vi "Fieldbus Read_Write.vi"(8 "error in (no error)":errorcluster, 11 "FHPP in":refnum<class "FHPP.lvclass">) -> (0 "error out":errorcluster, 3 "FHPP out":refnum<class "FHPP.lvclass">)   [LabVIEW 2022 SP3, in "FHPP.lvclass"]
uses:
  FHPP.lvclass
  FHPP.lvclass/FHPP.ctl
  <vilib>/Modbus/master/Modbus Master.lvclass
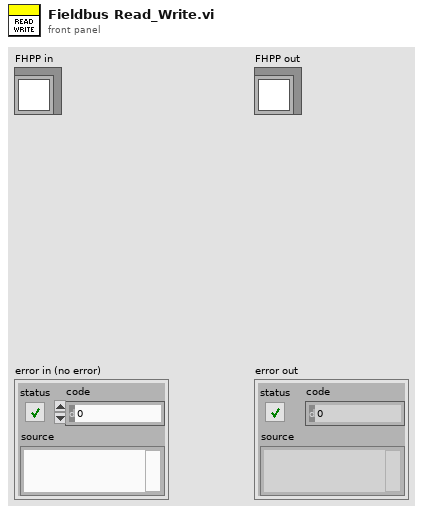
[diagram p1: front panel]
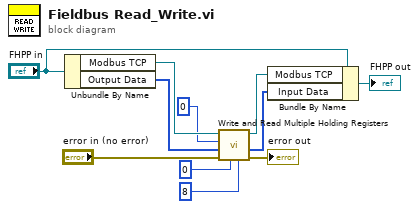
[diagram p0: block diagram]
diagram:
  n1 = Unbundle By Name("FHPP in") -> ("Modbus TCP"=w8:refnum<class "Modbus Master.lvclass">, "Output Data"=w7:u16[])
  n2 = call-dynamic "Write and Read Multiple Holding Registers.vi"("read count"=u16 8 ("number of holding registers"), "read operation starting address"=u16 0, "error in (no error)"="error in (no error)", "values to write"=w7, "write operation starting address"=u16 0, "Modbus master in"=w8) -> ("error out"=→"error out":errorcluster, "values read"=w9:u16[], "Modbus master out"=w11:refnum<class "Modbus Master.lvclass">)  [unwired: 3 in]
  n3 = Bundle By Name(cluster="FHPP in", "Modbus TCP"=w11, "Input Data"=w9) -> (→"FHPP out":refnum<class "FHPP.lvclass">)
